vi "resource read.vi"(8 "error in":errorcluster, 10 "id":i32, 11 "message json":string) -> (0 "error out":errorcluster, 3 "response":string)   [LabVIEW 2025, in "MCP Server.lvlib"]
uses:
  MCP Server.lvlib
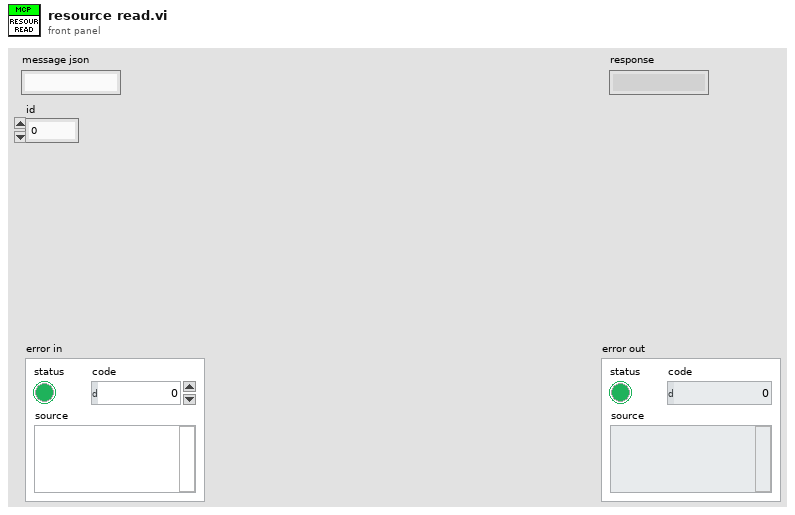
[diagram p1: front panel]
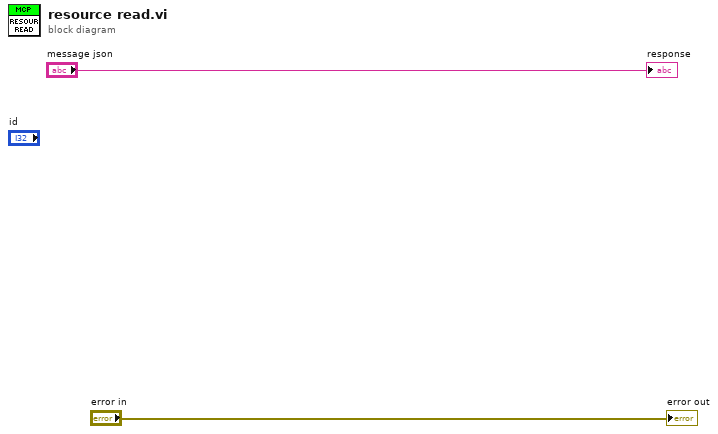
[diagram p0: block diagram]
diagram:
  "error out" <- "error in"
  "response" <- "message json"
